vi "configure_approach.vi"() -> ()   [LabVIEW 2020, in "Coarse Approach.lvclass"]
uses:
  Coarse Approach.lvclass
panel:
  in  "Setpoint ratio":dbl
  out "error out":errorcluster
  in  "error in":errorcluster
  out "Coarse Approach out":refnum<class "Coarse Approach.lvclass">
  in  "Coarse Approach in":refnum<class "Coarse Approach.lvclass">
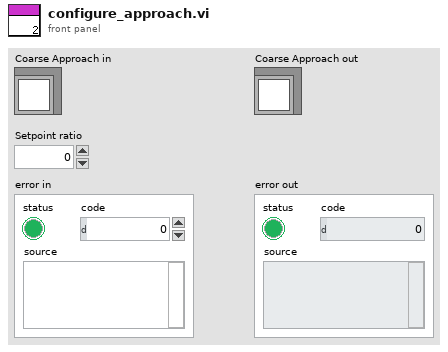
[diagram p1: front panel]
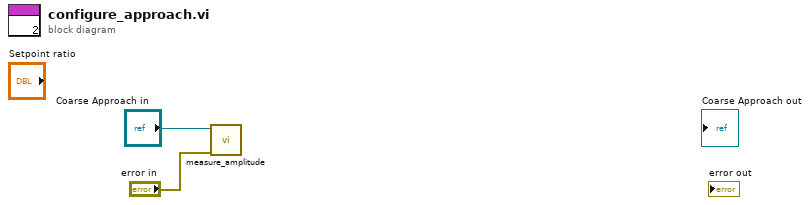
[diagram p0: block diagram]
diagram:
  n1 = call "measure_amplitude.vi"("error in"="error in", "Coarse Approach in"="Coarse Approach in") -> ()  [unwired: 6 in, 4 out]
